vi "First Code Point.vi"(11 "String":string) -> (3 "First Code Point":u32)   [LabVIEW 2020, in "Stream.lvlib" / "URLPattern.lvclass"]
uses:
  URLPattern.lvclass
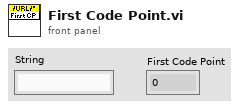
[diagram p1: front panel]
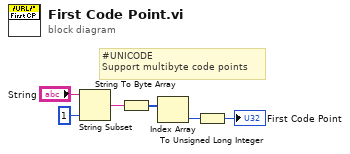
[diagram p0: block diagram]
diagram:
  # "#UNICODE\nSupport multibyte code points"
  n1 = String Subset(string="String", length (rest)=1 ("length (rest)")) -> (substring=w4:string)  [unwired: 1 in]
  n2 = String To Byte Array(string=w4) -> (unsigned byte array=w3:u8[])
  n3 = Index Array(array=w3) -> (element=w2:u8)  [unwired: 1 in]
  n4 = To Unsigned Long Integer(number=w2) -> (unsigned 32bit integer=→"First Code Point":u32)
